vi "RotationScaling(TEST).vi"(4 "binning":i16=1, 8 "Active Cursor":u32, 9 "Angle":dbl=0.2644720085068628 format="%.2f", 10 "GuideGraph":refnum<vi>, 11 "GuidePixScale":dbl=0.323 format="%.2f") -> (0 "Y":i16=481, 3 "X":i16=421)   [LabVIEW 2011]
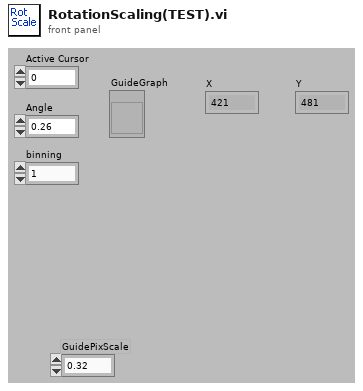
[diagram p1: front panel]
types:
  T1 = typedef "LVRangeTypeDef.ctl" = cluster{"Minimum":dbl, "Maximum":dbl, "Increment":dbl, "Minor Increment":dbl, "Start":dbl}
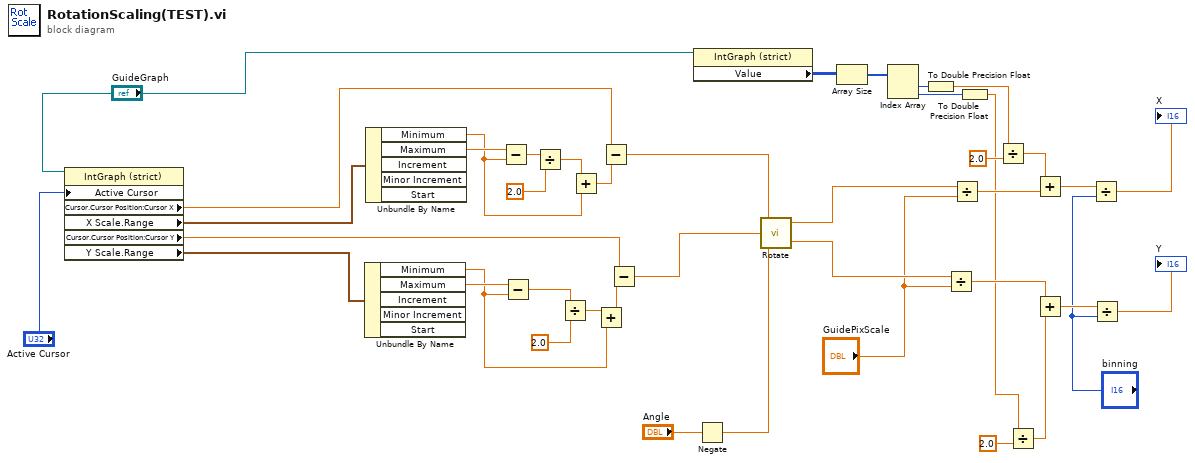
[diagram p0: block diagram]
diagram:
  n1 = property on="Property Node" class="IntGraph (strict)"(reference="GuideGraph", "Active Cursor"="Active Cursor") -> ("Cursor.Cursor Position:Cursor X"=w37:dbl, "X Scale.Range"=w38:T1, "Cursor.Cursor Position:Cursor Y"=w36:dbl, "Y Scale.Range"=w41:T1)  [unwired: 1 in, 2 out]
  n2 = Unbundle By Name(w41) -> ("Minimum"=w23:dbl, "Maximum"=w39:dbl)  [unwired: 3 out]
  n3 = Unbundle By Name(w38) -> ("Minimum"=w26:dbl, "Maximum"=w40:dbl)  [unwired: 3 out]
  n4 = Subtract(x=w40, y=w26) -> (x-y=w33:dbl)
  n5 = Subtract(x=w39, y=w23) -> (x-y=w30:dbl)
  n6 = Divide(x=w33, y=2.0) -> (x/y=w25:dbl)
  n7 = Divide(x=w30, y=2.0) -> (x/y=w22:dbl)
  n8 = Add(x=w25, y=w26) -> (x+y=w24:dbl)
  n9 = Add(x=w22, y=w23) -> (x+y=w21:dbl)
  n10 = Subtract(x=w37, y=w24) -> (x-y=w35:dbl)
  n11 = Subtract(x=w36, y=w21) -> (x-y=w34:dbl)
  n12 = property class="IntGraph (strict)"(reference="GuideGraph") -> ("Value"=w6:u32[][])  [unwired: 1 in, 2 out]
  n13 = Negate(x="Angle") -> (-x=w13:dbl)
  n14 = call "Rotate.vi"("Angle(rad)"=w13, "Y"=w34, "X"=w35) -> ("rotY"=w28:dbl, "rotX"=w29:dbl)
  n15 = Array Size(array=w6) -> (size(s)=w5:i32[])
  n16 = Index Array(array=w5) -> (element #1=w4:i32, element #2=w3:i32)  [unwired: 2 in]
  n17 = To Double Precision Float(number=w4) -> (double precision float=w2:dbl)
  n18 = Divide(x=w28, y="GuidePixScale") -> (x/y=w18:dbl)
  n19 = Divide(x=w29, y="GuidePixScale") -> (x/y=w16:dbl)
  n20 = To Double Precision Float(number=w3) -> (double precision float=w1:dbl)
  n21 = Divide(x=w2, y=2.0) -> (x/y=w15:dbl)
  n22 = Divide(x=w1, y=2.0) -> (x/y=w17:dbl)
  n23 = Add(x=w15, y=w16) -> (x+y=w11:dbl)
  n24 = Add(x=w18, y=w17) -> (x+y=w12:dbl)
  n25 = Divide(x=w11, y="binning") -> (x/y=→"X":dbl)
  n26 = Divide(x=w12, y="binning") -> (x/y=→"Y":dbl)
